vi "FormSystemSet.vi"() -> ()   [LabVIEW 2012]
uses:
  S7Ref.vi
panel:
  out "XY Graph 12":T1(graph) caption="空载测定曲线"
  in  "通道":enum16{"", "输入轴", "输出轴小量程", "输出轴大量程"}(ring)
  in  "标定":bool
  in  "传感器参数":string[][](table)
  out "读取成功":bool
  in  "添加":bool
  in  "标定 2":bool
  in  "缩放系数":dbl
  in  "实际输入":dbl
  in  "标定点数":string[][](table)
  in  "流量标定":bool
  in  "实际体积":dbl
  in  "缩放系数 2":dbl
  in  "缩放系数 1":dbl
  out "mm":dbl[](array[numeric])
  in  "偏移量":dbl
  in  "确定":bool
  # "inputMoveSpeed"
  # "mm/s"
  # "outputMoveSpeed"
  # "mm/s"
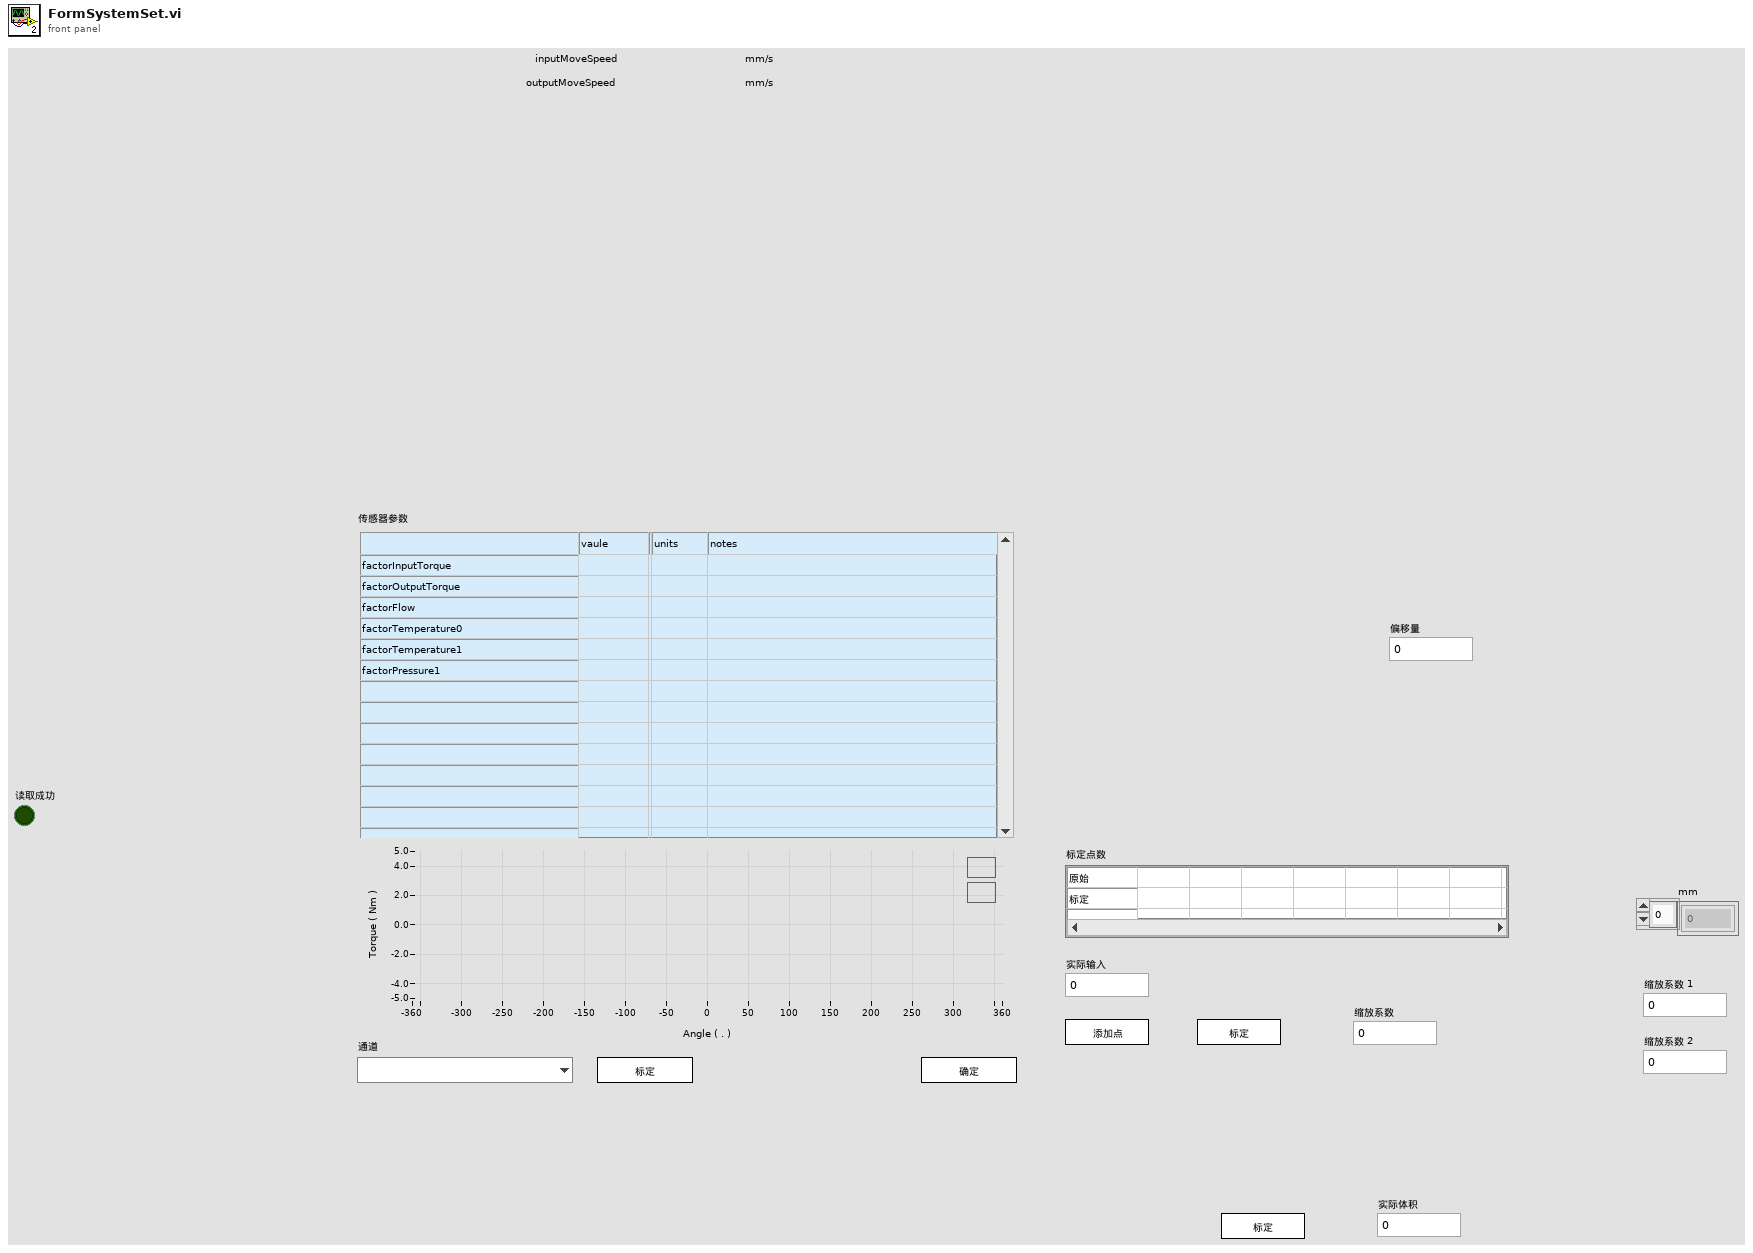
[diagram p1: front panel]
types:
  T1 = cluster{"Array of Single":sgl[], "Array of Single":sgl[]}[]
  T2 = enum8{"Enabled", "Disabled", "Disabled and Grayed Out"}
  T3 = cluster{"userCode":string, "userName":string, "userStatus":string, "connectionMode":string, "takesTime":string, "countDone":string, "countOK":string, "countNG":string, "rigStatus":string, "productsName":string, "partCode1":string, "partCode2":string, "partCode3":string}
  T4 = cluster{"A":dbl[], "B":dbl[], "C":dbl[], "D":dbl[]}
  T5 = cluster{"vaule":dbl, "vaule":dbl, "limitL":dbl, "limitL":dbl}
  T6 = cluster{"max":dbl, "min":dbl, "uripp":dbl, "average":dbl}
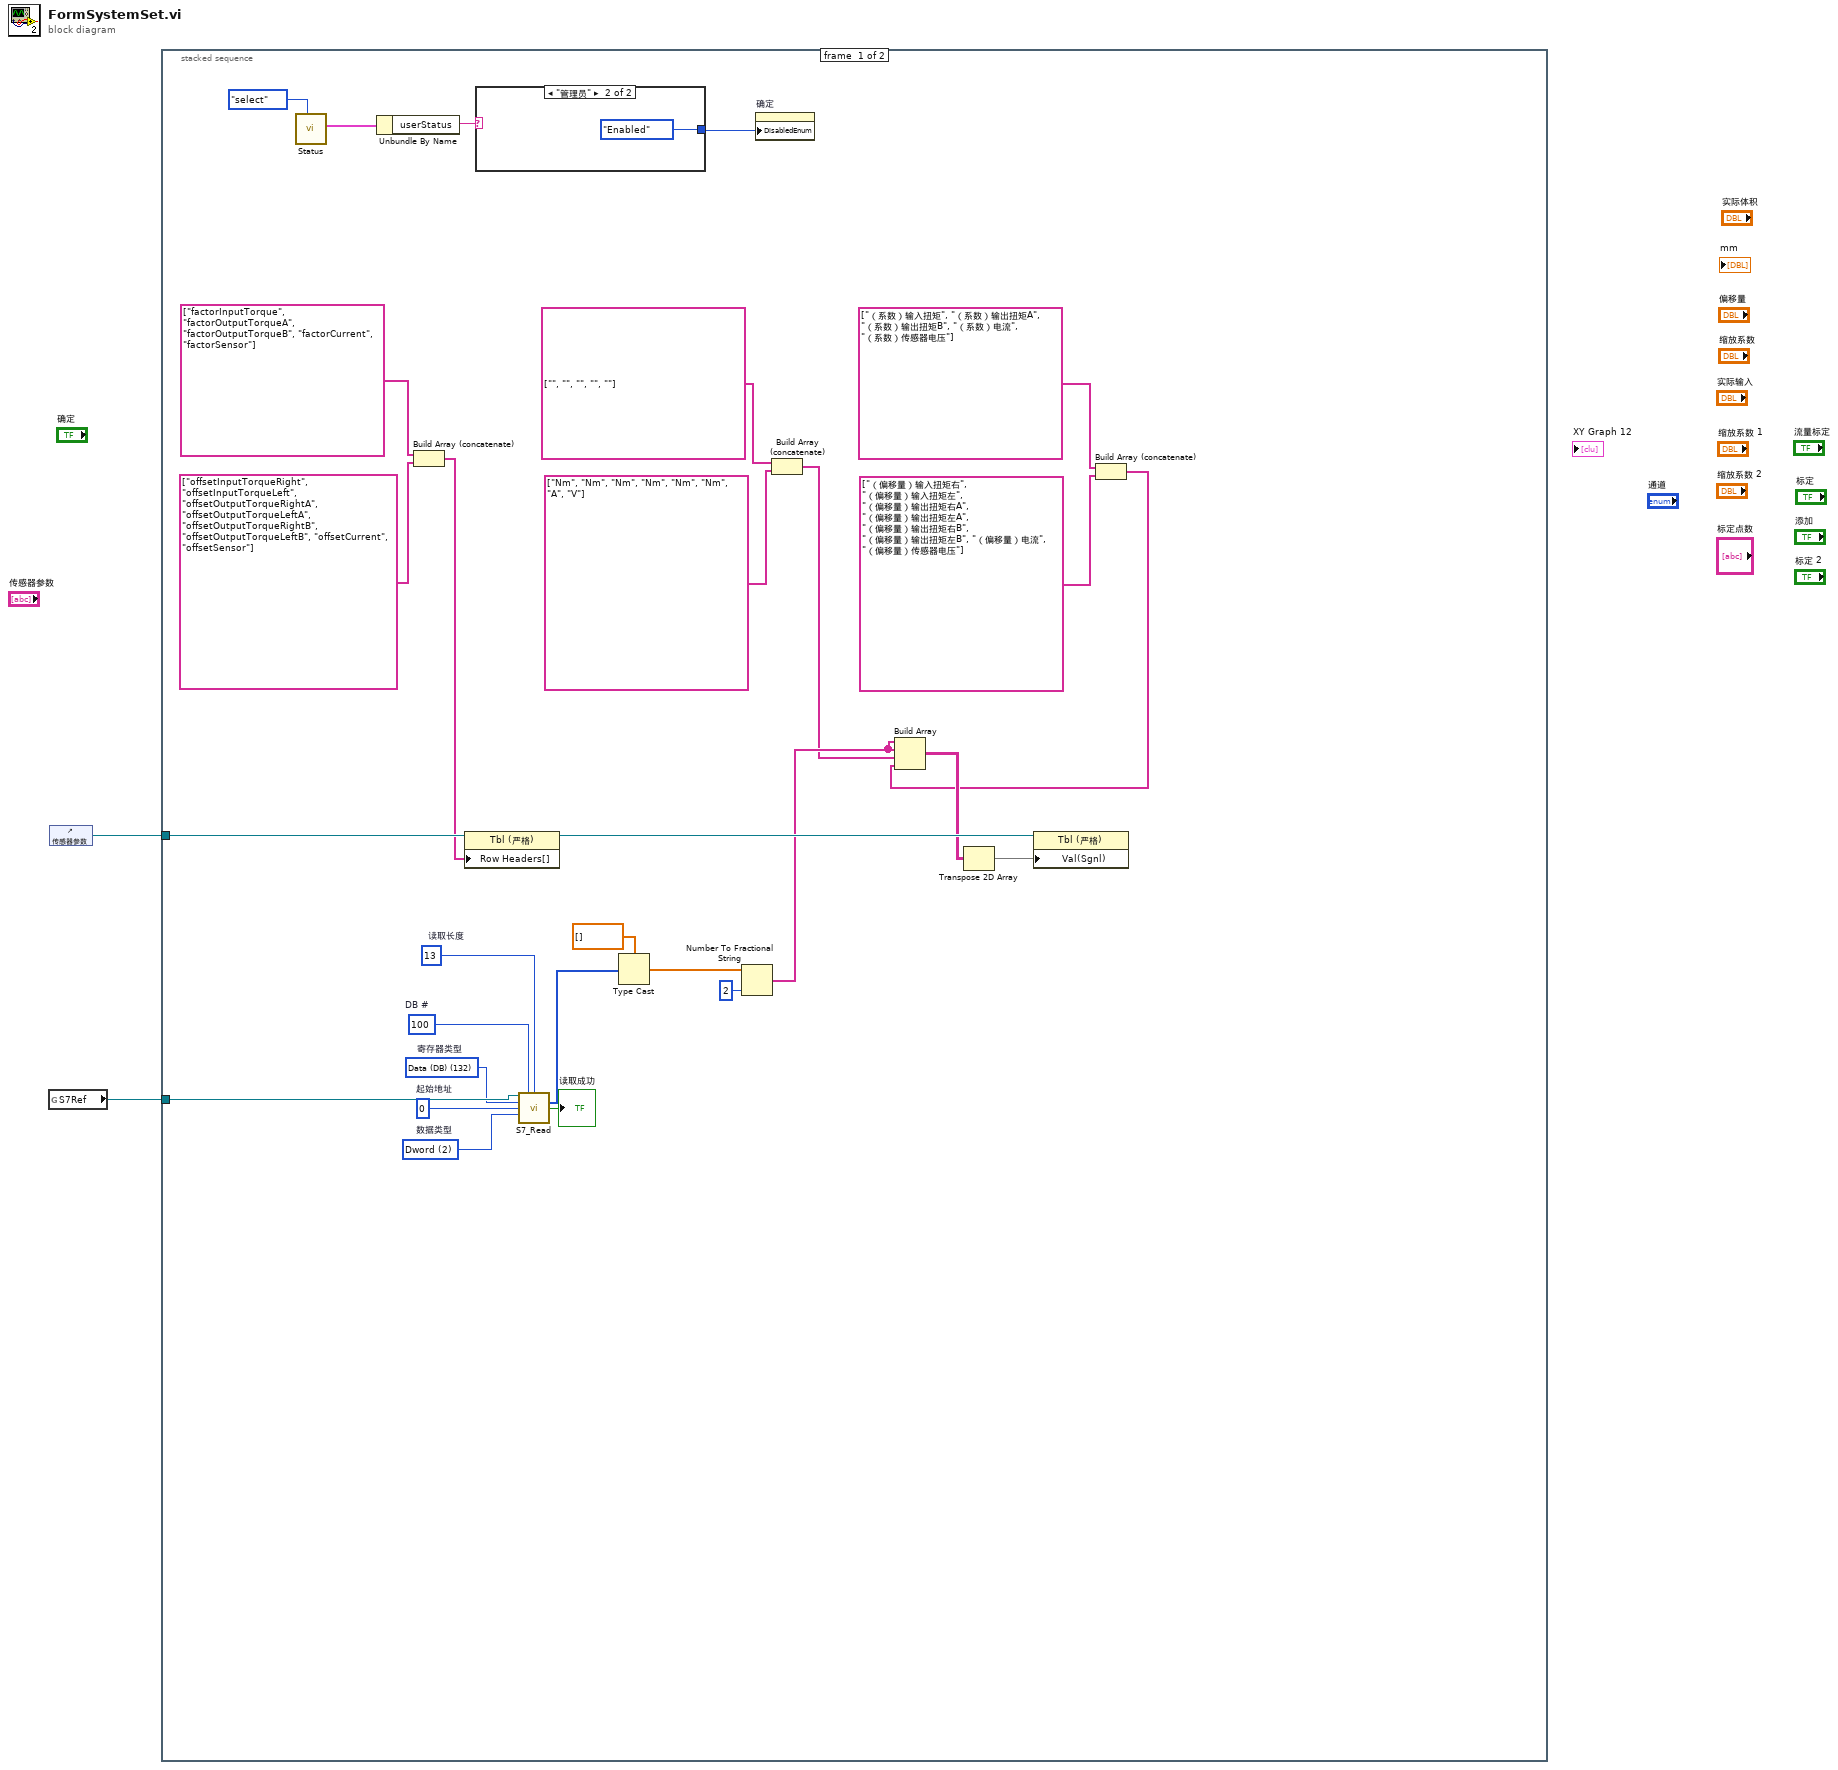
[diagram p0: block diagram]
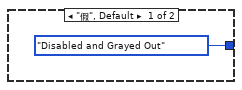
[diagram p2: hidden frame]
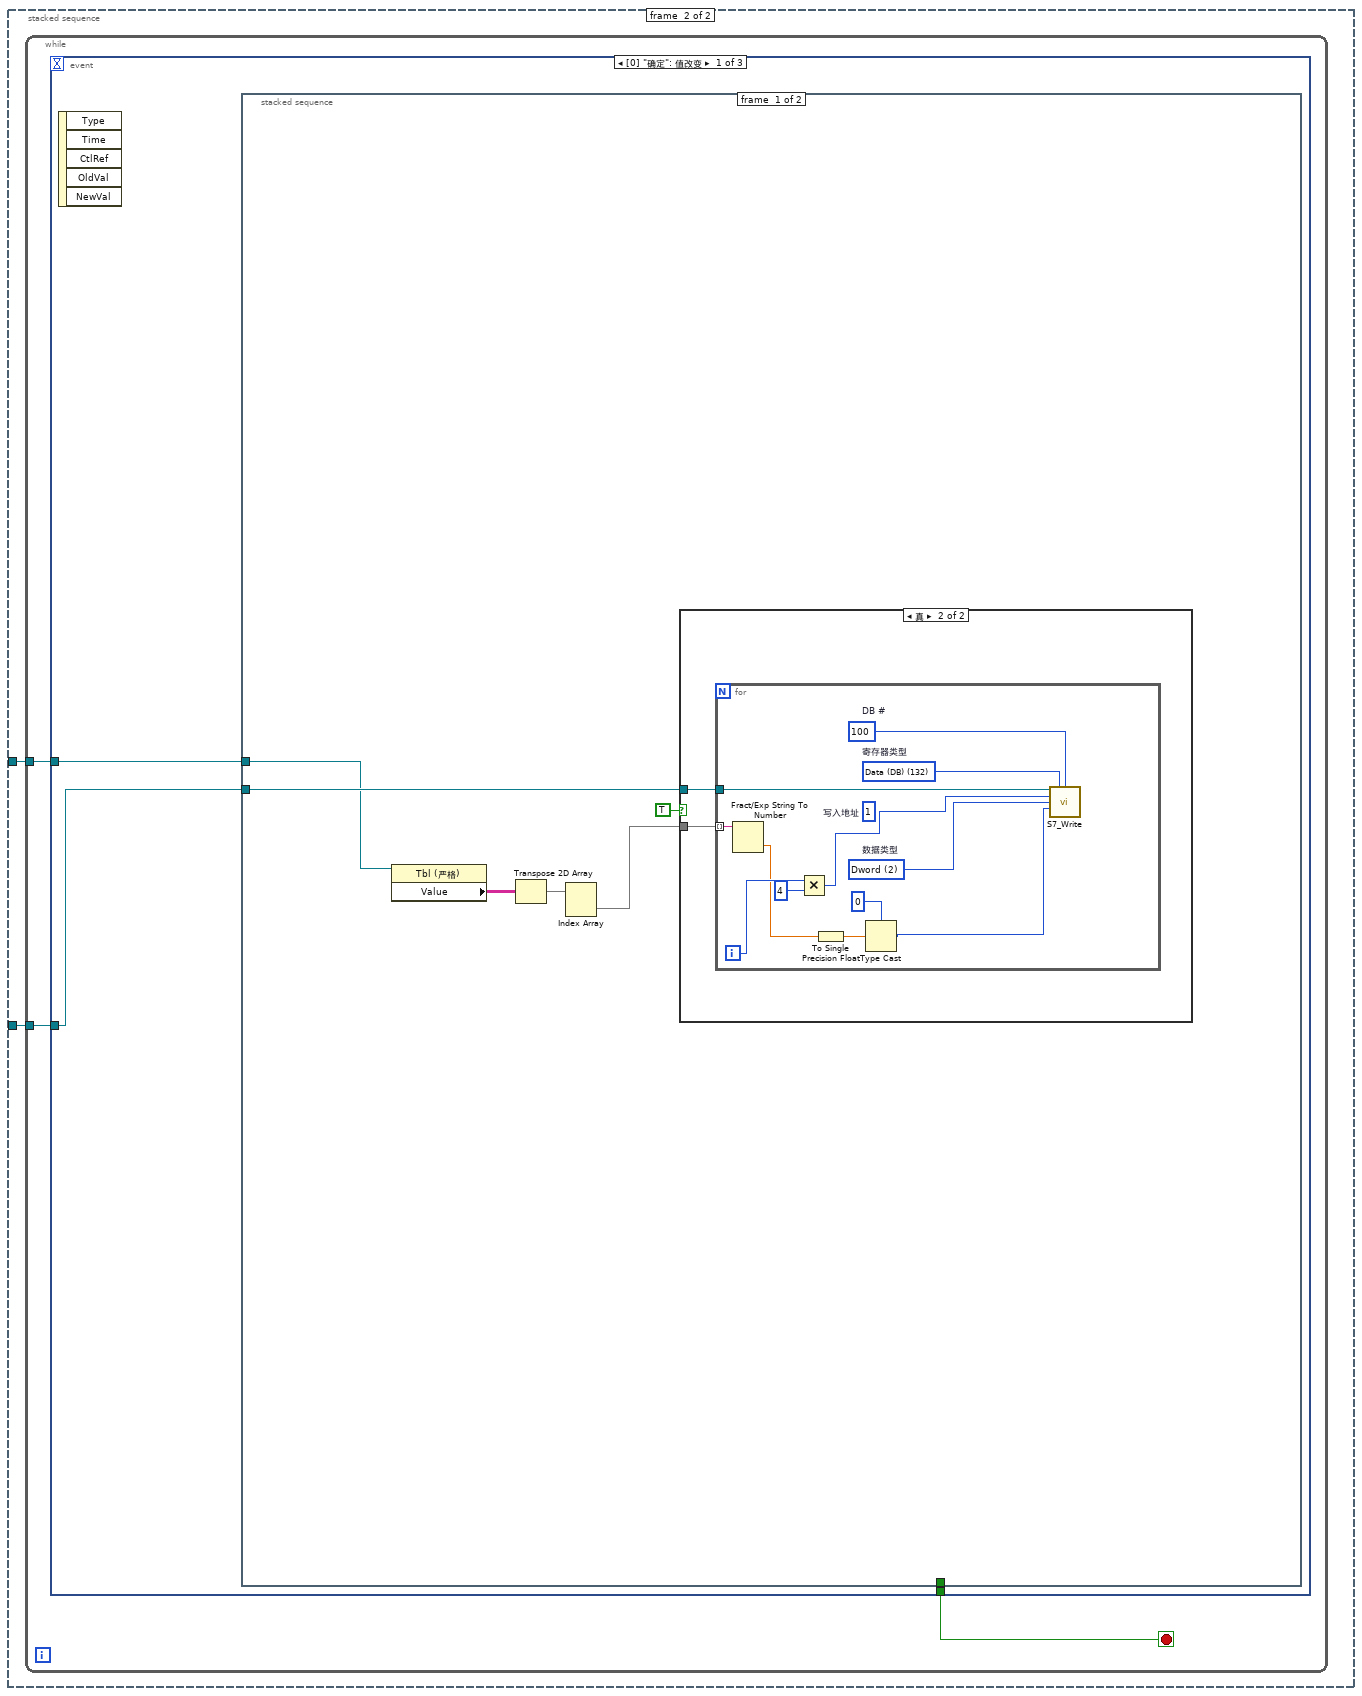
[diagram p3: hidden frame]
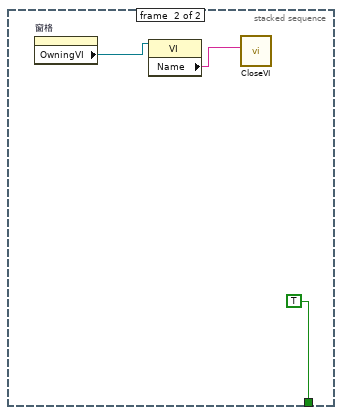
[diagram p5: hidden frame]
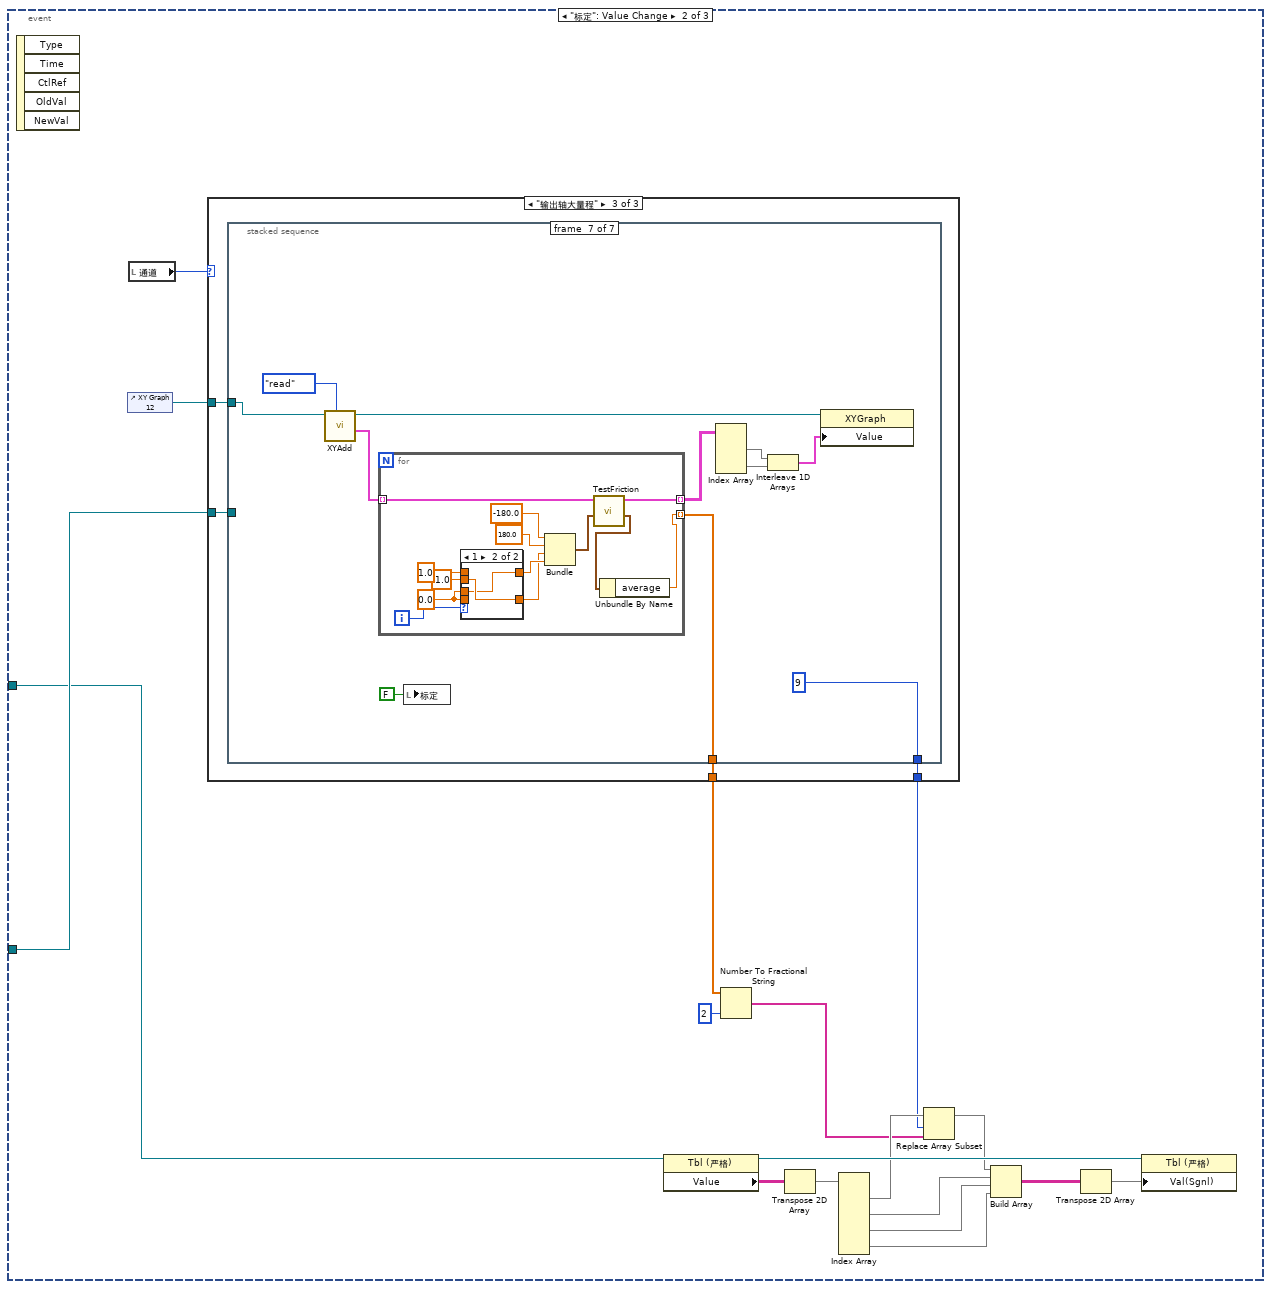
[diagram p6: hidden frame]
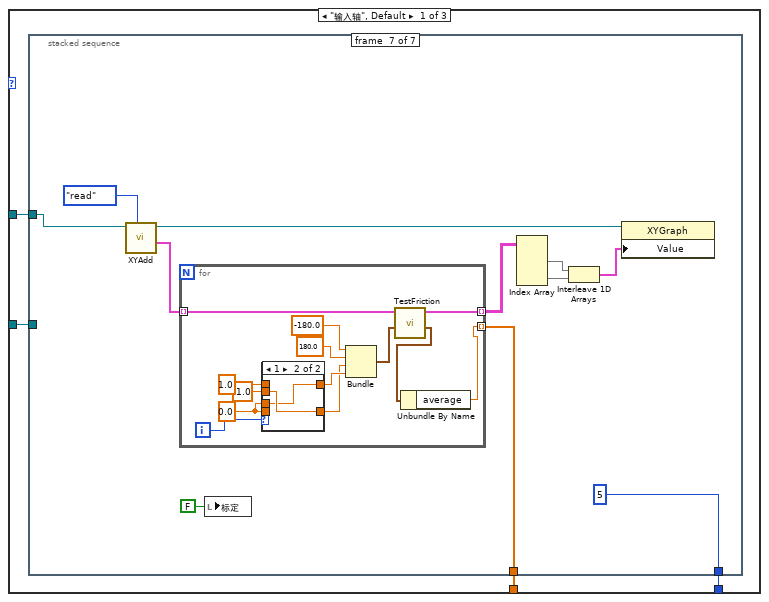
[diagram p7: hidden frame]
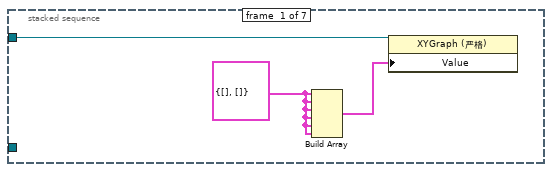
[diagram p8: hidden frame]
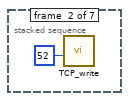
[diagram p9: hidden frame]
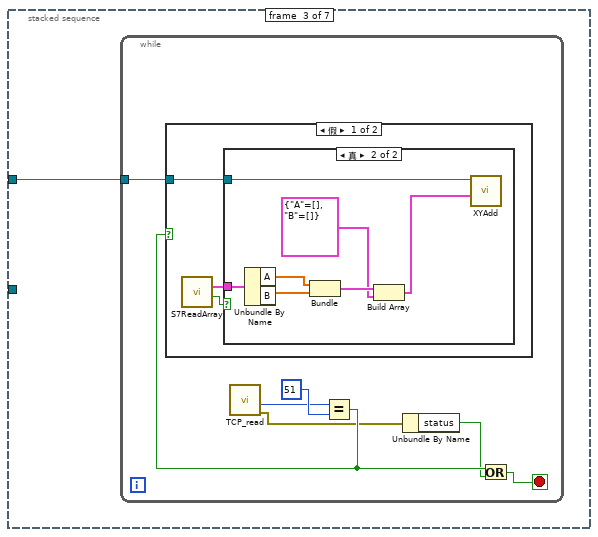
[diagram p10: hidden frame]
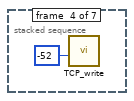
[diagram p13: hidden frame]
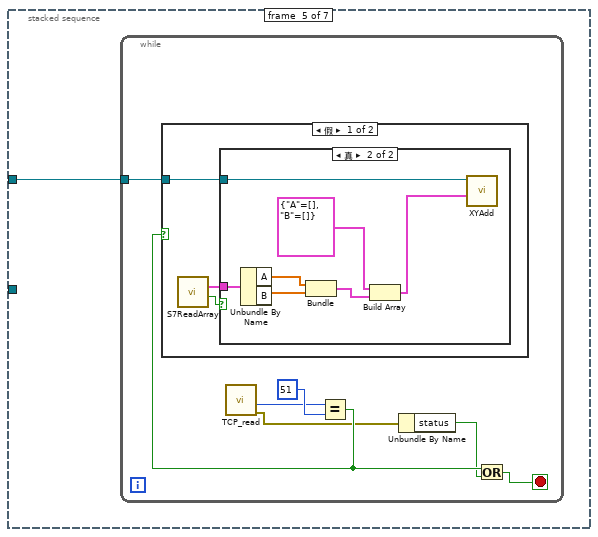
[diagram p14: hidden frame]
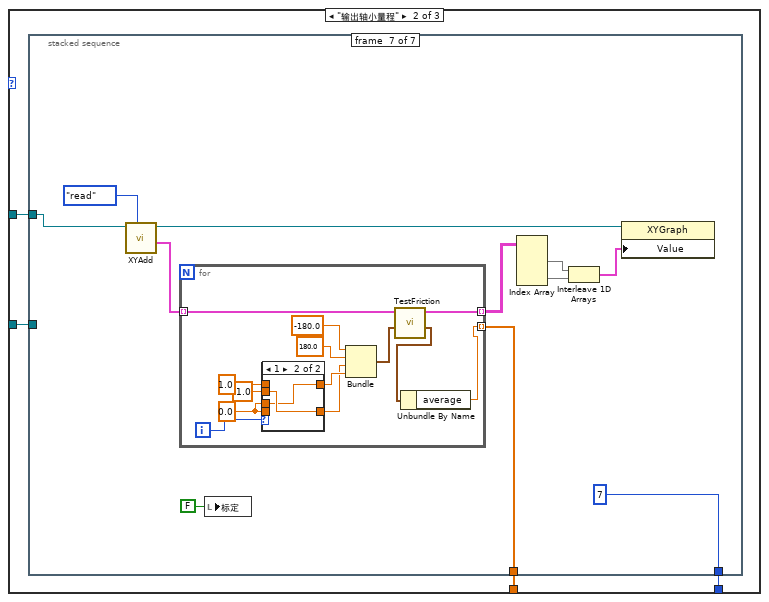
[diagram p19: hidden frame]
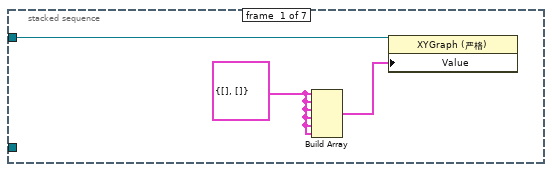
[diagram p20: hidden frame]
diagram:
  n1 = global read "S7Ref.vi" "S7Ref"() -> (w2:refnum<k5>)
  n2 = control-ref of="传感器参数"() -> (w1:refnum<vi>)
  n3 = stacked-sequence {
    tunnel: w2 -> [w31 w35]
    tunnel: w1 -> [w18 w34]
    frame #0 {
      w24 = u16 100  # DB #
      w27 = u16 2 items=["byte", "word", "Dword"]  # 数据类型
      w28 = u32 0  # 起始地址
      w29 = u8 132 items=["I/O (P)"=128, "Input (I)"=129, "Output (Q)"=130, "Bit Memory (M)"=131, "Data (DB)"=132, "Instance Data (DI)"=133, "Local Data (L)"=134, "Predecessor Local Data (VL)"=135]  # 寄存器类型
      w26 = u16 13  # 读取长度
      n4 = call "Status.vi"("模式"=enum16{"select", "insert", "update", "delete"}."select") -> ("元素"=w21:T3)  [unwired: 10 in]
      n5 = Unbundle By Name(w21) -> ("userStatus"=w22:string)
      n6 = Build Array (concatenate)(string[] ["factorInputTorque", "factorOutputTorqueA", "factorOutputTorqueB", "factorCurrent", "factorSensor"] ("添加的数组"), string[] ["offsetInputTorqueRight", "offsetInputTorqueLeft", "offsetOutputTorqueRightA", "offsetOutputTorqueLeftA", "offsetOutputTorqueRightB", "offsetOutputTorqueLeftB", "offsetCurrent", "offsetSensor"] ("添加的数组")) -> (w9:string[])
      n7 = property class="Tbl (严格)"(reference=w18, "Row Headers[]"=w9) -> (reference out=w17:refnum<vi>)  [unwired: 1 in, 1 out]
      n8 = case shown="\"管理员\"" w22 {
        tunnel: [T2."Disabled and Grayed Out" ("禁用") T2."Enabled" ("禁用")] -> w19
        frame "假", Default {
        }
        frame "管理员" {
        }
      }
      n9 = call "S7_Read.vi"("TCP"=w31, "DB #"=w24, "读取长度"=w26, "寄存器类型"=w29, "起始地址"=w28, "数据类型"=w27) -> ("数据"=w25:u32[], "读取成功"=→"读取成功":bool)  [unwired: 6 in, 2 out]
      n10 = Type Cast(type=sgl[] [] ("添加的数组"), x=w25) -> (*(type *) &x=w16:sgl[])
      n11 = Number To Fractional String(number=w16, precision (6)=i16 2 ("精度(6)")) -> (F-format string=w12:string[])  [unwired: 2 in]
      n12 = property on="确定" class="Bool"("DisabledEnum"=w19) -> ()  [unwired: 2 in, 2 out]
      n13 = Build Array (concatenate)(string[] ["", "", "", "", ""] ("添加的数组"), string[] ["Nm", "Nm", "Nm", "Nm", "Nm", "Nm", "A", "V"] ("添加的数组")) -> (w6:string[])
      n14 = Build Array (concatenate)(string[] ["（系数）输入扭矩", "（系数）输出扭矩A", "（系数）输出扭矩B", "（系数）电流", "（系数）传感器电压"] ("添加的数组"), string[] ["（偏移量）输入扭矩右", "（偏移量）输入扭矩左", "（偏移量）输出扭矩右A", "（偏移量）输出扭矩左A", "（偏移量）输出扭矩右B", "（偏移量）输出扭矩左B", "（偏移量）电流", "（偏移量）传感器电压"] ("添加的数组")) -> (w3:string[])
      n15 = Build Array(w12, w12, w6, w3) -> (w14:string[][])
      n16 = Transpose 2D Array(2D array=w14) -> (transposed array=w13:string[][])
      n17 = property class="Tbl (严格)"(reference=w17, "Val(Sgnl)"=w13) -> ()  [unwired: 1 in, 2 out]
    }
    frame #1 {
      n18 = while {
        tunnel: w35 -> [w37]
        tunnel: w34 -> [w36]
        stop <- w38 stop-if-true
        n19 = event shown="[0] \"确定\": 值改变" {
          selector: _ -> [_ _ _]
          dyn-events: _ -> [_ _ _]
          timeout: _ -> [_ _ _]
          tunnel: [w41 _ TRUE] -> w38
          tunnel: w37 -> [w40 w81 _]
          tunnel: w36 -> [w39 w67 _]
          event "确定": Value Change {
            n20 = event-data() -> ()  [unwired: 1 in, 5 out]
            n21 = stacked-sequence {
              tunnel: [_ TRUE] -> w41
              tunnel: w40 -> [w47 _]
              tunnel: w39 -> [w46 _]
              frame #0 {
                n22 = property class="Tbl (严格)"(reference=w46) -> ("Value"=w44:string[][])  [unwired: 1 in, 2 out]
                n23 = Transpose 2D Array(2D array=w44) -> (transposed array=w43:string[][])
                n24 = Index Array(array=w43) -> (element=w45:string[])  [unwired: 2 in]
                n25 = case shown="真" TRUE {
                  tunnel: w47 -> [_ w49]
                  tunnel: w45 -> [_ w48]
                  frame False {
                  }
                  frame True {
                    n26 = for {
                      tunnel: w49 -> [w57]
                      tunnel: w48 -> [w51] mode=indexing
                      i -> [w56]
                      w60 = u16 2 items=["byte", "word", "Dword"]  # 数据类型
                      (unwired) u32 1  # 写入地址
                      w59 = u16 100  # DB #
                      w61 = u8 132 items=["I/O (P)"=128, "Input (I)"=129, "Output (Q)"=130, "Bit Memory (M)"=131, "Data (DB)"=132, "Instance Data (DI)"=133, "Local Data (L)"=134, "Predecessor Local Data (VL)"=135]  # 寄存器类型
                      n27 = Fract/Exp String To Number(string=w51) -> (number=w50:dbl)  [unwired: 3 in, 1 out]
                      n28 = Multiply(x=w56, y=4) -> (x*y=w54:i32)
                      n29 = To Single Precision Float(number=w50) -> (single precision float=w52:sgl)
                      n30 = Type Cast(type=u32 0, x=w52) -> (*(type *) &x=w53:u32)
                      n31 = call "S7_Write.vi"("TCP"=w57, "寄存器类型"=w61, "DB #"=w59, "写入地址"=w54, "数据类型"=w60, "写入数据"=w53) -> ()  [unwired: 7 in, 3 out]
                    }
                  }
                }
              }
              frame #1 {
                n32 = property on="窗格" class="Pane"() -> ("OwningVI"=w62:refnum<vi>)  [unwired: 2 in, 2 out]
                n33 = property on="属性节点" class="VI"(reference=w62) -> ("Name"=w63:string)  [unwired: 1 in, 2 out]
                n34 = call "CloseVI.vi"("名称或相对路径"=w63) -> ()  [unwired: 10 in, 1 out]
              }
            }
          }
          event "标定": Value Change {
            n35 = event-data() -> ()  [unwired: 1 in, 5 out]
            n36 = control-ref of="XY Graph 12"() -> (w80:refnum<vi>)
            n37 = local read "通道"() -> (w82:enum16{"", "输入轴", "输出轴小量程", "输出轴大量程"})
            n38 = case shown="\"输出轴大量程\"" w82 {
              tunnel: w81 -> [w86 w159 w232]
              tunnel: w80 -> [w85 w158 w231]
              tunnel: [w84 w157 w230] -> w66
              tunnel: [w83 w156 w229] -> w65
              frame "输入轴", Default {
                n39 = stacked-sequence {
                  tunnel: w86 -> [_ _ _ _ _ _ _]
                  tunnel: w85 -> [w87 _ w91 _ w110 _ w131]
                  tunnel: [_ _ _ _ _ _ w129] -> w84
                  tunnel: [_ _ _ _ _ _ 5 ("索引")] -> w83
                  frame #0 {
                    w89 = cluster{dbl[], dbl[]} {[], []}
                    n40 = Build Array(w89, w89, w89, w89, w89, w89) -> (w88:cluster{dbl[], dbl[]}[])
                    n41 = property class="XYGraph (严格)"(reference=w87, "Value"=w88) -> ()  [unwired: 1 in, 2 out]
                  }
                  frame #1 {
                    n42 = call "TCP_write.vi"("写入数据"=i8 52) -> ()  [unwired: 11 in]
                  }
                  frame #2 {
                    n43 = while {
                      tunnel: w91 -> [w97]
                      stop <- w98 stop-if-true
                      n44 = call "TCP_read.vi"() -> ("error out"=w93:errorcluster, "元素"=w95:i8)  [unwired: 10 in]
                      n45 = Equal?(x=w95, y=i8 51) -> (x = y?=w94:bool)
                      n46 = case shown="假" w94 {
                        tunnel: w97 -> [w100 _]
                        frame False {
                          n47 = call "S7ReadArray.vi"() -> ("yes"=w99:bool, "输出簇"=w101:T4)  [unwired: 9 in, 1 out]
                          n48 = case shown="真" w99 {
                            tunnel: w101 -> [_ w103]
                            tunnel: w100 -> [_ w102]
                            frame False {
                            }
                            frame True {
                              n49 = Unbundle By Name(w103) -> ("A"=w108:dbl[], "B"=w107:dbl[])
                              n50 = Bundle("A"=w108, "B"=w107) -> (w105:cluster{"A":dbl[], "B":dbl[]})  [unwired: 1 in]
                              n51 = Build Array(w105, cluster{"A":dbl[], "B":dbl[]} {"A"=[], "B"=[]} ("元素")) -> (w106:cluster{"A":dbl[], "B":dbl[]}[])
                              n52 = call "XYAdd.vi"("数据"=w106, "XYGraph"=w102) -> ()  [unwired: 8 in, 2 out]
                            }
                          }
                        }
                        frame True {
                        }
                      }
                      n53 = Unbundle By Name(w93) -> ("status"=w92:bool)
                      n54 = Or(x=w94, y=w92) -> (x .or. y?=w98:bool)
                    }
                  }
                  frame #3 {
                    n55 = call "TCP_write.vi"("写入数据"=i8 -52) -> ()  [unwired: 11 in]
                  }
                  frame #4 {
                    n56 = while {
                      tunnel: w110 -> [w112]
                      stop <- w111 stop-if-true
                      n57 = call "TCP_read.vi"() -> ("error out"=w114:errorcluster, "元素"=w116:i8)  [unwired: 10 in]
                      n58 = Equal?(x=w116, y=i8 51) -> (x = y?=w115:bool)
                      n59 = case shown="假" w115 {
                        tunnel: w112 -> [w119 _]
                        frame False {
                          n60 = call "S7ReadArray.vi"() -> ("yes"=w118:bool, "输出簇"=w120:T4)  [unwired: 9 in, 1 out]
                          n61 = case shown="真" w118 {
                            tunnel: w120 -> [_ w124]
                            tunnel: w119 -> [_ w123]
                            frame False {
                            }
                            frame True {
                              n62 = Unbundle By Name(w124) -> ("A"=w127:dbl[], "B"=w126:dbl[])
                              n63 = Bundle("A"=w127, "B"=w126) -> (w121:cluster{"A":dbl[], "B":dbl[]})  [unwired: 1 in]
                              n64 = Build Array(cluster{"A":dbl[], "B":dbl[]} {"A"=[], "B"=[]} ("元素"), w121) -> (w125:cluster{"A":dbl[], "B":dbl[]}[])
                              n65 = call "XYAdd.vi"("数据"=w125, "XYGraph"=w123) -> ()  [unwired: 8 in, 2 out]
                            }
                          }
                        }
                        frame True {
                        }
                      }
                      n66 = Unbundle By Name(w114) -> ("status"=w113:bool)
                      n67 = Or(x=w115, y=w113) -> (x .or. y?=w111:bool)
                    }
                  }
                  frame #5 {
                  }
                  frame #6 {
                    n68 = call "XYAdd.vi"("枚举"=enum16{"add", "read", "reset"}."read", "XYGraph"=w131) -> ("XYData"=w137:cluster{dbl[], dbl[]}[], "XYGraph 2"=w138:refnum<vi>)  [unwired: 8 in]
                    n69 = for {
                      tunnel: w137 -> [w151] mode=indexing
                      tunnel: [w139] -> w129 mode=indexing
                      tunnel: [w144] -> w135 mode=indexing
                      i -> [w147]
                      w141 = 0.0 ("limitL")
                      n70 = case shown="1" w147 {
                        tunnel: 1.0 ("limitH") -> [w153 _]
                        tunnel: [w153 w154] -> w146
                        tunnel: w141 -> [w152 _]
                        tunnel: [w152 w155] -> w145
                        tunnel: -1.0 ("limitL") -> [_ w155]
                        tunnel: w141 -> [_ w154]
                        frame 0, Default {
                        }
                        frame 1 {
                        }
                      }
                      n71 = Bundle("vaule"=-180.0, "vaule"=180.0, "limitL"=w145, "limitL"=w146) -> (w150:T5)  [unwired: 1 in]
                      n72 = call "TestFriction.vi"("边界配置"=w150, "原始曲线"=w151) -> ("运算值"=w140:T6, "曲线数组"=w144:cluster{"X":dbl[], "Y":dbl[]}[])  [unwired: 8 in]
                      n73 = Unbundle By Name(w140) -> ("average"=w139:dbl)
                    }
                    n74 = local write "标定"(FALSE ("标定")) -> ()
                    n75 = Index Array(array=w135) -> (element #1=w132:cluster{"X":dbl[], "Y":dbl[]}[], element #2=w133:cluster{"X":dbl[], "Y":dbl[]}[])  [unwired: 4 in]
                    n76 = Interleave 1D Arrays(w132, w133) -> (w134:cluster{"X":dbl[], "Y":dbl[]}[])
                    n77 = property class="XYGraph"(reference=w138, "Value"=w134) -> ()  [unwired: 1 in, 2 out]
                  }
                }
              }
              frame "输出轴小量程" {
                n78 = stacked-sequence {
                  tunnel: w159 -> [_ _ _ _ _ _ _]
                  tunnel: w158 -> [w160 _ w164 _ w183 _ w204]
                  tunnel: [_ _ _ _ _ _ w202] -> w157
                  tunnel: [_ _ _ _ _ _ 7 ("索引")] -> w156
                  frame #0 {
                    w162 = cluster{dbl[], dbl[]} {[], []}
                    n79 = Build Array(w162, w162, w162, w162, w162, w162) -> (w161:cluster{dbl[], dbl[]}[])
                    n80 = property class="XYGraph (严格)"(reference=w160, "Value"=w161) -> ()  [unwired: 1 in, 2 out]
                  }
                  frame #1 {
                    n81 = call "TCP_write.vi"("写入数据"=i8 62) -> ()  [unwired: 11 in]
                  }
                  frame #2 {
                    n82 = while {
                      tunnel: w164 -> [w170]
                      stop <- w171 stop-if-true
                      n83 = call "TCP_read.vi"() -> ("error out"=w166:errorcluster, "元素"=w168:i8)  [unwired: 10 in]
                      n84 = Equal?(x=w168, y=i8 61) -> (x = y?=w167:bool)
                      n85 = case shown="假" w167 {
                        tunnel: w170 -> [w173 _]
                        frame False {
                          n86 = call "S7ReadArray.vi"() -> ("yes"=w172:bool, "输出簇"=w174:T4)  [unwired: 9 in, 1 out]
                          n87 = case shown="真" w172 {
                            tunnel: w174 -> [_ w176]
                            tunnel: w173 -> [_ w175]
                            frame False {
                            }
                            frame True {
                              n88 = Unbundle By Name(w176) -> ("A"=w181:dbl[], "B"=w180:dbl[])
                              n89 = Bundle("A"=w181, "B"=w180) -> (w178:cluster{"A":dbl[], "B":dbl[]})  [unwired: 1 in]
                              n90 = Build Array(w178, cluster{"A":dbl[], "B":dbl[]} {"A"=[], "B"=[]} ("元素")) -> (w179:cluster{"A":dbl[], "B":dbl[]}[])
                              n91 = call "XYAdd.vi"("数据"=w179, "XYGraph"=w175) -> ()  [unwired: 8 in, 2 out]
                            }
                          }
                        }
                        frame True {
                        }
                      }
                      n92 = Unbundle By Name(w166) -> ("status"=w165:bool)
                      n93 = Or(x=w167, y=w165) -> (x .or. y?=w171:bool)
                    }
                  }
                  frame #3 {
                    n94 = call "TCP_write.vi"("写入数据"=i8 -62) -> ()  [unwired: 11 in]
                  }
                  frame #4 {
                    n95 = while {
                      tunnel: w183 -> [w185]
                      stop <- w184 stop-if-true
                      n96 = call "TCP_read.vi"() -> ("error out"=w187:errorcluster, "元素"=w189:i8)  [unwired: 10 in]
                      n97 = Equal?(x=w189, y=i8 61) -> (x = y?=w188:bool)
                      n98 = case shown="假" w188 {
                        tunnel: w185 -> [w192 _]
                        frame False {
                          n99 = call "S7ReadArray.vi"() -> ("yes"=w191:bool, "输出簇"=w193:T4)  [unwired: 9 in, 1 out]
                          n100 = case shown="真" w191 {
                            tunnel: w193 -> [_ w197]
                            tunnel: w192 -> [_ w196]
                            frame False {
                            }
                            frame True {
                              n101 = Unbundle By Name(w197) -> ("A"=w200:dbl[], "B"=w199:dbl[])
                              n102 = Bundle("A"=w200, "B"=w199) -> (w194:cluster{"A":dbl[], "B":dbl[]})  [unwired: 1 in]
                              n103 = Build Array(cluster{"A":dbl[], "B":dbl[]} {"A"=[], "B"=[]} ("元素"), w194) -> (w198:cluster{"A":dbl[], "B":dbl[]}[])
                              n104 = call "XYAdd.vi"("数据"=w198, "XYGraph"=w196) -> ()  [unwired: 8 in, 2 out]
                            }
                          }
                        }
                        frame True {
                        }
                      }
                      n105 = Unbundle By Name(w187) -> ("status"=w186:bool)
                      n106 = Or(x=w188, y=w186) -> (x .or. y?=w184:bool)
                    }
                  }
                  frame #5 {
                  }
                  frame #6 {
                    n107 = call "XYAdd.vi"("枚举"=enum16{"add", "read", "reset"}."read", "XYGraph"=w204) -> ("XYData"=w210:cluster{dbl[], dbl[]}[], "XYGraph 2"=w211:refnum<vi>)  [unwired: 8 in]
                    n108 = for {
                      tunnel: w210 -> [w224] mode=indexing
                      tunnel: [w212] -> w202 mode=indexing
                      tunnel: [w217] -> w208 mode=indexing
                      i -> [w220]
                      w214 = 0.0 ("limitL")
                      n109 = case shown="1" w220 {
                        tunnel: 1.0 ("limitH") -> [w226 _]
                        tunnel: [w226 w227] -> w219
                        tunnel: w214 -> [w225 _]
                        tunnel: [w225 w228] -> w218
                        tunnel: -1.0 ("limitL") -> [_ w228]
                        tunnel: w214 -> [_ w227]
                        frame 0, Default {
                        }
                        frame 1 {
                        }
                      }
                      n110 = Bundle("vaule"=-180.0, "vaule"=180.0, "limitL"=w218, "limitL"=w219) -> (w223:T5)  [unwired: 1 in]
                      n111 = call "TestFriction.vi"("边界配置"=w223, "原始曲线"=w224) -> ("运算值"=w213:T6, "曲线数组"=w217:cluster{"X":dbl[], "Y":dbl[]}[])  [unwired: 8 in]
                      n112 = Unbundle By Name(w213) -> ("average"=w212:dbl)
                    }
                    n113 = local write "标定"(FALSE ("标定")) -> ()
                    n114 = Index Array(array=w208) -> (element #1=w205:cluster{"X":dbl[], "Y":dbl[]}[], element #2=w206:cluster{"X":dbl[], "Y":dbl[]}[])  [unwired: 4 in]
                    n115 = Interleave 1D Arrays(w205, w206) -> (w207:cluster{"X":dbl[], "Y":dbl[]}[])
                    n116 = property class="XYGraph"(reference=w211, "Value"=w207) -> ()  [unwired: 1 in, 2 out]
                  }
                }
              }
              frame "输出轴大量程" {
                n117 = stacked-sequence {
                  tunnel: w232 -> [_ _ _ _ _ _ _]
                  tunnel: w231 -> [w233 _ w237 _ w256 _ w277]
                  tunnel: [_ _ _ _ _ _ w275] -> w230
                  tunnel: [_ _ _ _ _ _ 9 ("索引")] -> w229
                  frame #0 {
                    w235 = cluster{dbl[], dbl[]} {[], []}
                    n118 = Build Array(w235, w235, w235, w235, w235, w235) -> (w234:cluster{dbl[], dbl[]}[])
                    n119 = property class="XYGraph (严格)"(reference=w233, "Value"=w234) -> ()  [unwired: 1 in, 2 out]
                  }
                  frame #1 {
                    n120 = call "TCP_write.vi"("写入数据"=i8 63) -> ()  [unwired: 11 in]
                  }
                  frame #2 {
                    n121 = while {
                      tunnel: w237 -> [w243]
                      stop <- w244 stop-if-true
                      n122 = call "TCP_read.vi"() -> ("error out"=w239:errorcluster, "元素"=w241:i8)  [unwired: 10 in]
                      n123 = Equal?(x=w241, y=i8 61) -> (x = y?=w240:bool)
                      n124 = case shown="假" w240 {
                        tunnel: w243 -> [w246 _]
                        frame False {
                          n125 = call "S7ReadArray.vi"() -> ("yes"=w245:bool, "输出簇"=w247:T4)  [unwired: 9 in, 1 out]
                          n126 = case shown="真" w245 {
                            tunnel: w247 -> [_ w249]
                            tunnel: w246 -> [_ w248]
                            frame False {
                            }
                            frame True {
                              n127 = Unbundle By Name(w249) -> ("A"=w254:dbl[], "B"=w253:dbl[])
                              n128 = Bundle("A"=w254, "B"=w253) -> (w251:cluster{"A":dbl[], "B":dbl[]})  [unwired: 1 in]
                              n129 = Build Array(w251, cluster{"A":dbl[], "B":dbl[]} {"A"=[], "B"=[]} ("元素")) -> (w252:cluster{"A":dbl[], "B":dbl[]}[])
                              n130 = call "XYAdd.vi"("数据"=w252, "XYGraph"=w248) -> ()  [unwired: 8 in, 2 out]
                            }
                          }
                        }
                        frame True {
                        }
                      }
                      n131 = Unbundle By Name(w239) -> ("status"=w238:bool)
                      n132 = Or(x=w240, y=w238) -> (x .or. y?=w244:bool)
                    }
                  }
                  frame #3 {
                    n133 = call "TCP_write.vi"("写入数据"=i8 -63) -> ()  [unwired: 11 in]
                  }
                  frame #4 {
                    n134 = while {
                      tunnel: w256 -> [w258]
                      stop <- w257 stop-if-true
                      n135 = call "TCP_read.vi"() -> ("error out"=w260:errorcluster, "元素"=w262:i8)  [unwired: 10 in]
                      n136 = Equal?(x=w262, y=i8 61) -> (x = y?=w261:bool)
                      n137 = case shown="假" w261 {
                        tunnel: w258 -> [w265 _]
                        frame False {
                          n138 = call "S7ReadArray.vi"() -> ("yes"=w264:bool, "输出簇"=w266:T4)  [unwired: 9 in, 1 out]
                          n139 = case shown="真" w264 {
                            tunnel: w266 -> [_ w270]
                            tunnel: w265 -> [_ w269]
                            frame False {
                            }
                            frame True {
                              n140 = Unbundle By Name(w270) -> ("A"=w273:dbl[], "B"=w272:dbl[])
                              n141 = Bundle("A"=w273, "B"=w272) -> (w267:cluster{"A":dbl[], "B":dbl[]})  [unwired: 1 in]
                              n142 = Build Array(cluster{"A":dbl[], "B":dbl[]} {"A"=[], "B"=[]} ("元素"), w267) -> (w271:cluster{"A":dbl[], "B":dbl[]}[])
                              n143 = call "XYAdd.vi"("数据"=w271, "XYGraph"=w269) -> ()  [unwired: 8 in, 2 out]
                            }
                          }
                        }
                        frame True {
                        }
                      }
                      n144 = Unbundle By Name(w260) -> ("status"=w259:bool)
                      n145 = Or(x=w261, y=w259) -> (x .or. y?=w257:bool)
                    }
                  }
                  frame #5 {
                  }
                  frame #6 {
                    n146 = call "XYAdd.vi"("枚举"=enum16{"add", "read", "reset"}."read", "XYGraph"=w277) -> ("XYData"=w283:cluster{dbl[], dbl[]}[], "XYGraph 2"=w284:refnum<vi>)  [unwired: 8 in]
                    n147 = for {
                      tunnel: w283 -> [w297] mode=indexing
                      tunnel: [w285] -> w275 mode=indexing
                      tunnel: [w290] -> w281 mode=indexing
                      i -> [w293]
                      w287 = 0.0 ("limitL")
                      n148 = case shown="1" w293 {
                        tunnel: 1.0 ("limitH") -> [w299 _]
                        tunnel: [w299 w300] -> w292
                        tunnel: w287 -> [w298 _]
                        tunnel: [w298 w301] -> w291
                        tunnel: -1.0 ("limitL") -> [_ w301]
                        tunnel: w287 -> [_ w300]
                        frame 0, Default {
                        }
                        frame 1 {
                        }
                      }
                      n149 = Bundle("vaule"=-180.0, "vaule"=180.0, "limitL"=w291, "limitL"=w292) -> (w296:T5)  [unwired: 1 in]
                      n150 = call "TestFriction.vi"("边界配置"=w296, "原始曲线"=w297) -> ("运算值"=w286:T6, "曲线数组"=w290:cluster{"X":dbl[], "Y":dbl[]}[])  [unwired: 8 in]
                      n151 = Unbundle By Name(w286) -> ("average"=w285:dbl)
                    }
                    n152 = local write "标定"(FALSE ("标定")) -> ()
                    n153 = Index Array(array=w281) -> (element #1=w278:cluster{"X":dbl[], "Y":dbl[]}[], element #2=w279:cluster{"X":dbl[], "Y":dbl[]}[])  [unwired: 4 in]
                    n154 = Interleave 1D Arrays(w278, w279) -> (w280:cluster{"X":dbl[], "Y":dbl[]}[])
                    n155 = property class="XYGraph"(reference=w284, "Value"=w280) -> ()  [unwired: 1 in, 2 out]
                  }
                }
              }
            }
            n156 = property class="Tbl (严格)"(reference=w67) -> (reference out=w72:refnum<vi>, "Value"=w73:string[][])  [unwired: 1 in, 1 out]
            n157 = Number To Fractional String(number=w66, precision (6)=i16 2 ("精度(6)")) -> (F-format string=w68:string[])  [unwired: 2 in]
            n158 = Transpose 2D Array(2D array=w73) -> (transposed array=w74:string[][])
            n159 = Index Array(array=w74) -> (element #1=w70:string[], element #2=w71:string[], element #3=w75:string[], element #4=w76:string[])  [unwired: 8 in]
            n160 = Replace Array Subset(array=w70, new element=w68, index=w65) -> (w69:string[])
            n161 = Build Array(w69, w71, w75, w76) -> (w78:string[][])
            n162 = Transpose 2D Array(2D array=w78) -> (transposed array=w77:string[][])
            n163 = property class="Tbl (严格)"(reference=w72, "Val(Sgnl)"=w77) -> ()  [unwired: 1 in, 2 out]
          }
          event Panel Close {
            n164 = event-data() -> ()  [unwired: 1 in, 3 out]
          }
        }
      }
    }
  }
